vi "overlay_generation.vi"(4 "center radius":dbl, 5 "Color":u32(colorbox)=16448250, 6 "number of rings":i32, 9 "Title":string, 10 "Image Src":T1, 11 "fringe preview on":bool) -> (3 "stream_overlay_out":T1)   [LabVIEW 2011]
doc: "Creates Overlay pattern to help with the alignment of the setup. The input image is copied and a new memory space is create to hold the overlay image in order to keep the originally created pattern."
uses:
  <vilib>/vision/Image Controls.llb/IMAQ Image.ctl
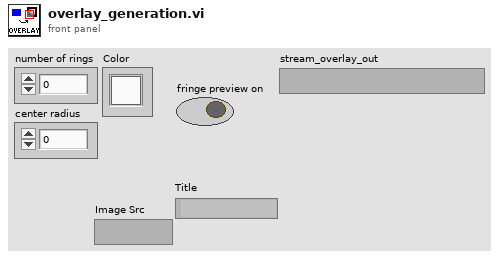
[diagram p1: front panel]
types:
  T1 = typedef "IMAQ Image.ctl" = refnum<image>
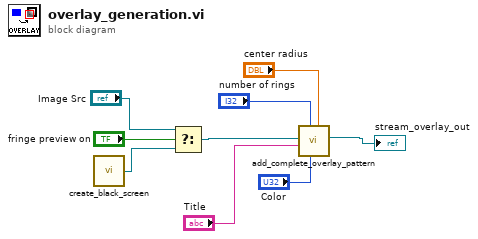
[diagram p0: block diagram]
diagram:
  n1 = call "create_black_screen.vi"() -> ("img_black_screen"=w8:T1)  [unwired: 5 in]
  n2 = Select(t="Image Src", s="fringe preview on", f=w8) -> (s? t:f=w6:T1)
  n3 = call "add_complete_overlay_pattern.vi"("center radius"="center radius", "Color"="Color", "number of rings"="number of rings", "Image Name"="Title", "Image Src"=w6) -> ("Image Out"=→"stream_overlay_out":T1)  [unwired: 6 in]
